vi "PXI_Host_I16_Write_NewMethod_Benchmark.vi"() -> ()   [LabVIEW 2018]
uses:
  <vilib>/Platform/TimedLoop/XDataNode/timing_clust.ctl
  <vilib>/Platform/TimedLoop/XDataNode/nitl_modes.ctl
  <vilib>/Platform/TimedLoop/XDataNode/wakeup.ctl
  cRIO RT/FPGA Bitfile Register Operations/Scalar IO Operations/Write Methods/Write Data Register/Instances/Write I16.vi
  cRIO RT/FPGA Bitfile Register Operations/Scalar IO Operations/Utilities/Find Register Offset.vi
  cRIO RT/FPGA Bitfile Register Operations/Scalar IO Operations/SubVIs/Check Register Data Store.vi
  cRIO RT/FPGA Bitfile Register Operations/Scalar IO Operations/Error Handling/Error 6001.vi
  cRIO RT/FPGA Bitfile Register Operations/Scalar IO Operations/Error Handling/Error 6000.vi
  cRIO RT/FPGA Bitfile Register Operations/Scalar IO Operations/Error Handling/Error 6002.vi
  cRIO RT/FPGA Bitfile Register Operations/Scalar IO Operations/Error Handling/Error 6006.vi
  <vilib>/FPGAPlugInAG/Dynamic/niLvFpga_Close_Dynamic.vi
  <vilib>/platform/TimedLoop/XDataNode/XDataNode.xnode
  <vilib>/rvi/interface/nirviCloseFPGA/nirviCloseFPGA.xnode
  cRIO RT/FPGA Bitfile Register Operations/Scalar IO Operations/FPGA Register IO.lvlib
  <vilib>/Platform/TimedLoop/XDataNode/XDNodeRunTimeDep.lvlib
panel:
  out "Maximum(s)":dbl
  out "Standard deviation":dbl
  out "Waveform Graph":dbl[](graph)
  out "error out":errorcluster
  out "Execution time (s)":dbl
  # "Recorded time"
  # "3.37551E-5"
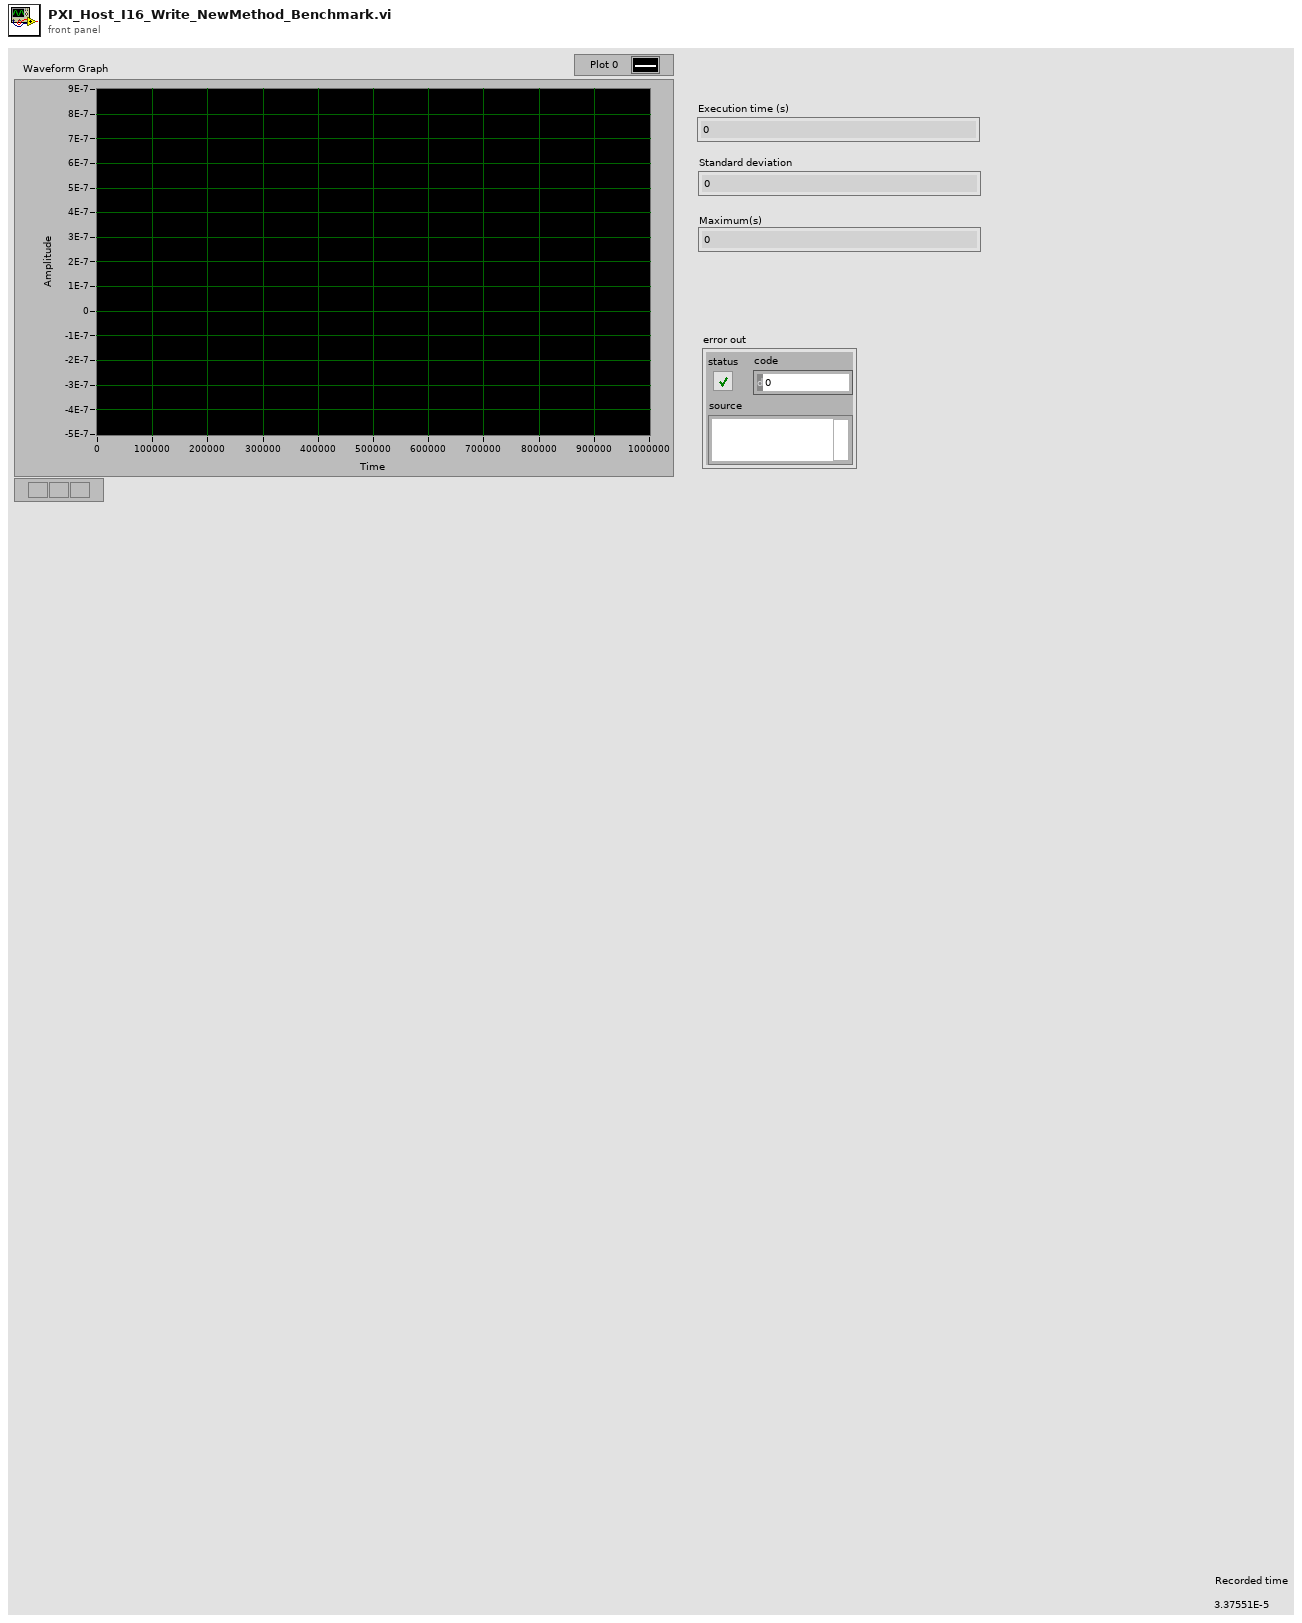
[diagram p1: front panel]
types:
  T1 = typedef "XDNodeRunTimeDep.lvlib/timing_clust.ctl" = cluster{"Expected End [f-1]":u64, "Actual End [f-1]":u64, "Finished Late? [f-1]":bool, "Expected End [i-1]":u64, "Actual End [i-1]":u64, "Finished Late? [i-1]":bool, "Expected Start [i]":u64, "Actual Start [i]":u64, "Expected Start [f]":u64, "Actual Start [f]":u64, "Source Name":string, "Structure Name":string, "Period":i64, "Deadline":i64, "Offset":i64, "Start":i64, "Priority":i32, "Timeout":i32, "Mode":T2, "Wakeup Reason":T3, "Error":errorcluster, "Source Type":string, "Secondary Source Type":string, "Global End Time":u64, "Global Start Time":u64, "Frame Duration":u64, "Iteration Duration":u64, "Assigned CPU":i32, "I/O Scan Engine Mode":u32}
  T2 = typedef "XDNodeRunTimeDep.lvlib/nitl_modes.ctl" = enum32{"No Change", "Process missed periods, maintain original phase", "Discard missed periods, maintain original phase", "Process missed periods, ignore original phase", "Discard missed periods, ignore original phase"}
  T3 = typedef "XDNodeRunTimeDep.lvlib/wakeup.ctl" = enum32{"Normal", "Aborted", "Asynchronous wakeup", "Timing source error", "Timed loop error", "Timeout"}
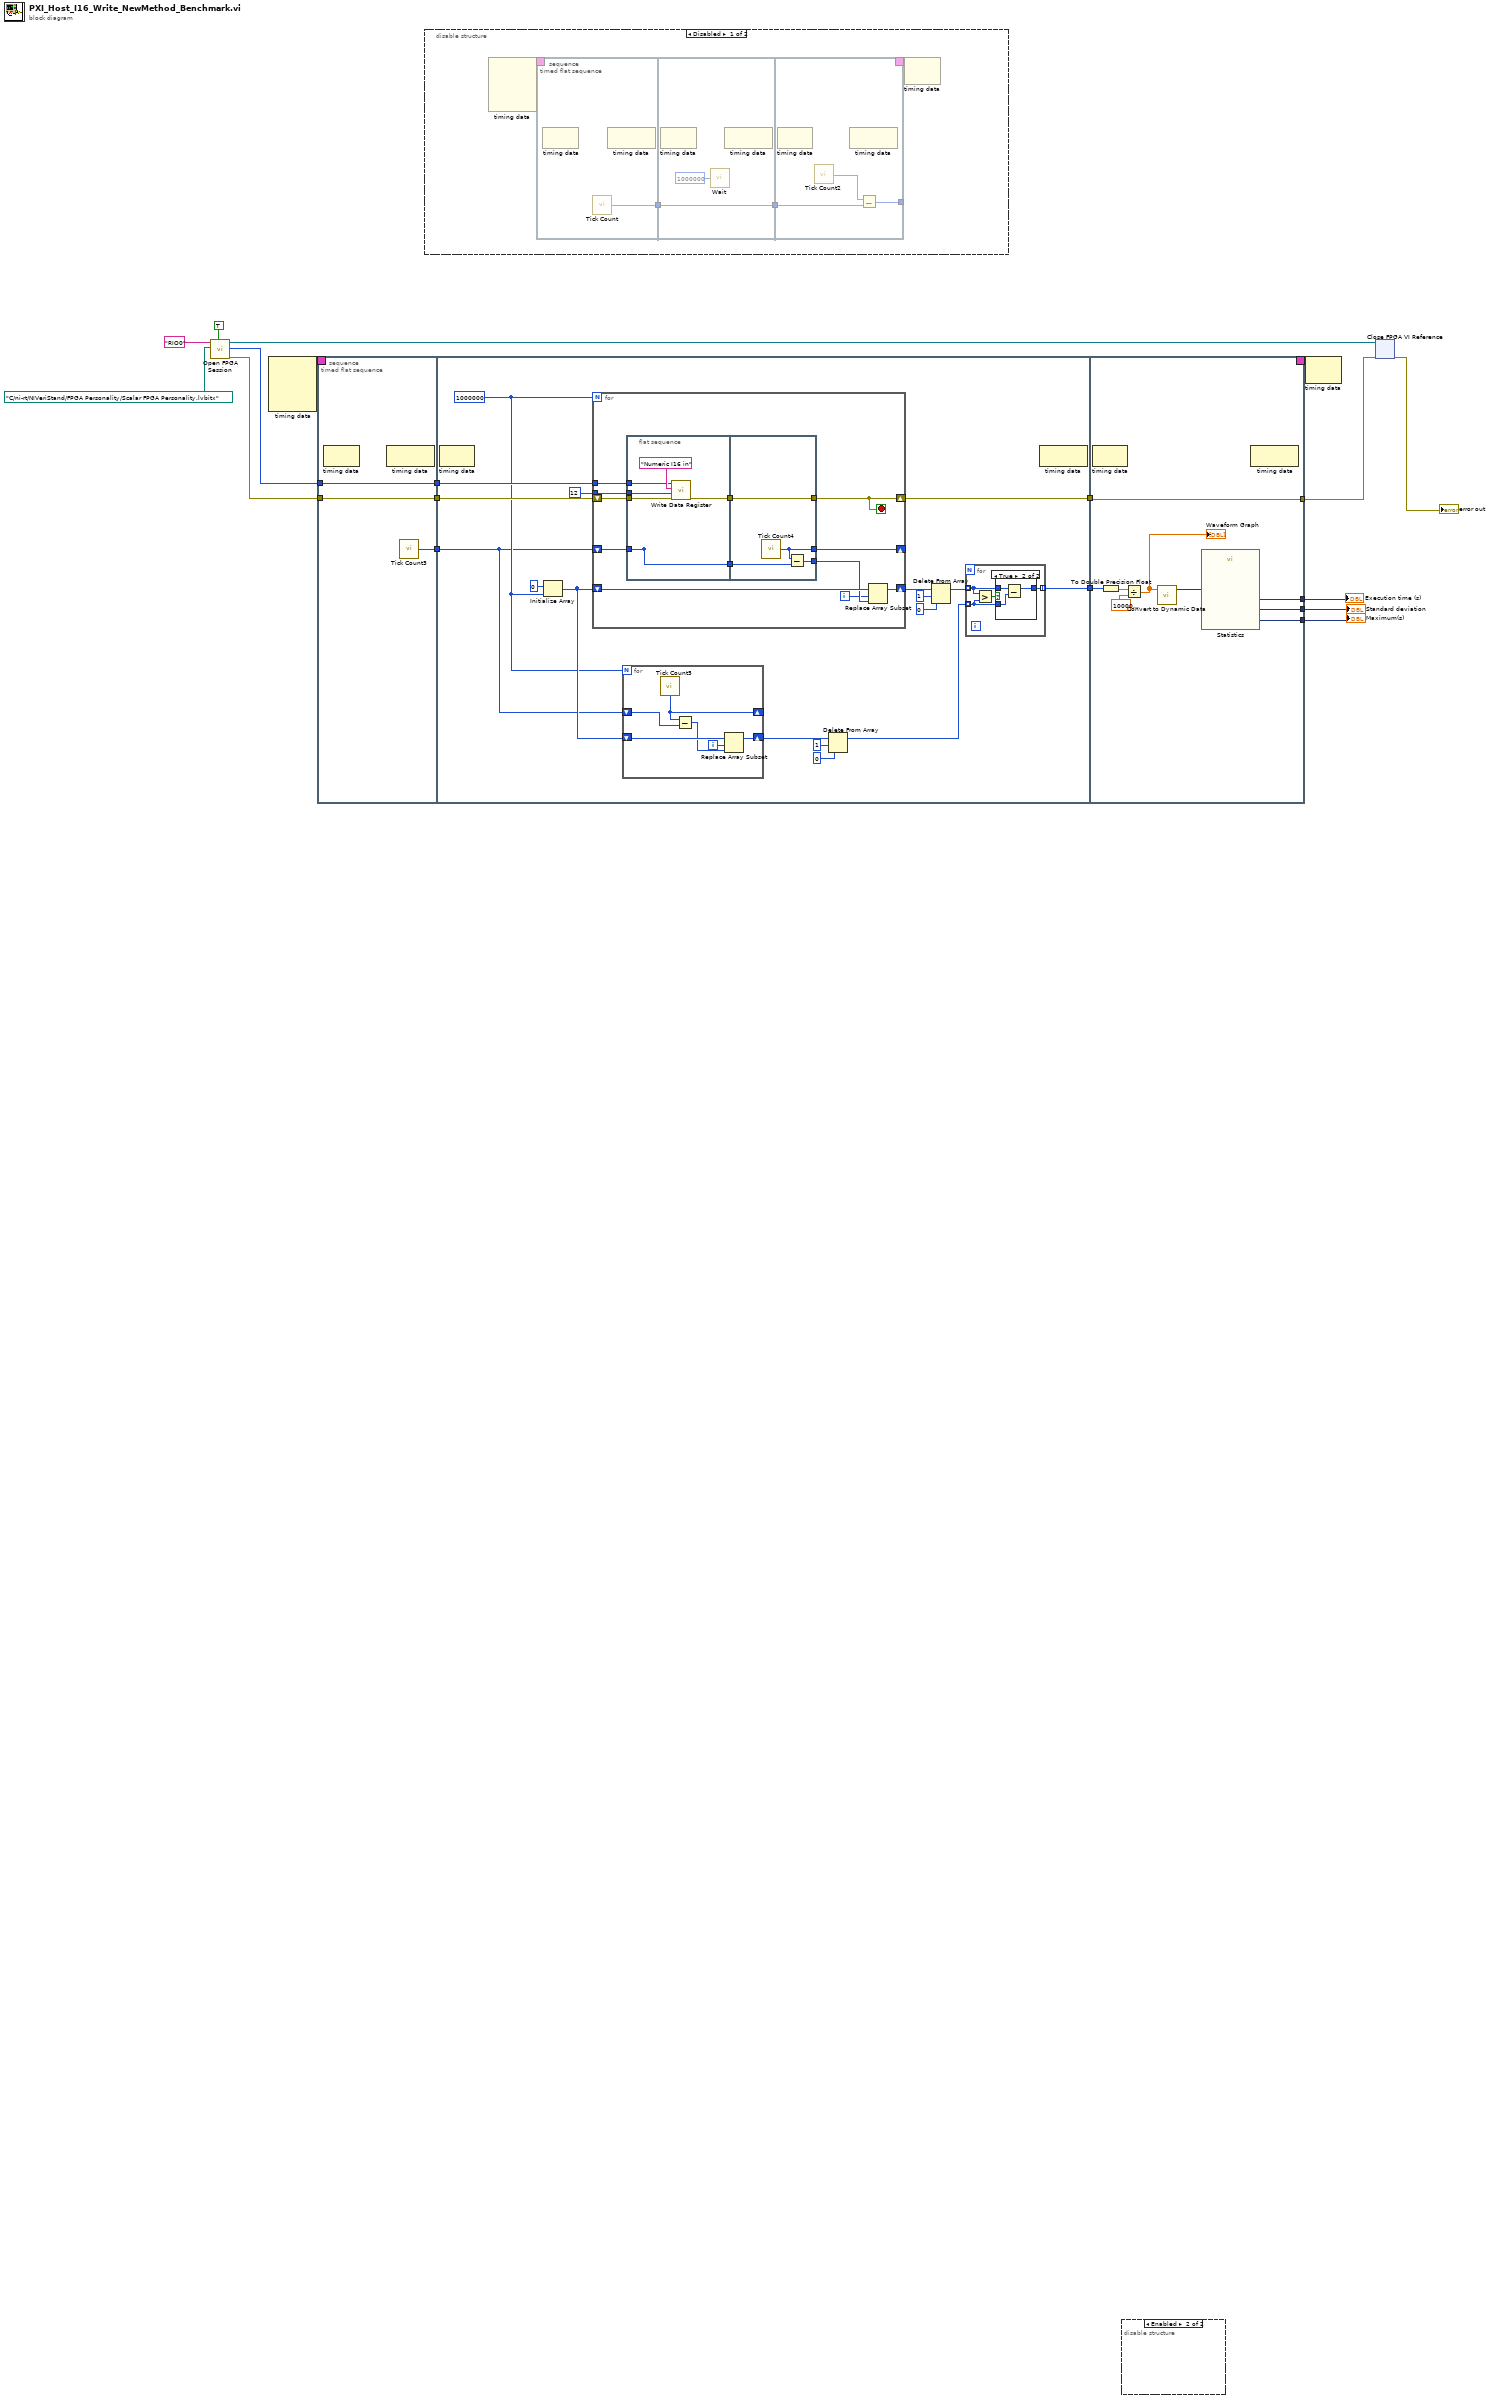
[diagram p0: block diagram]
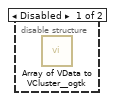
[diagram p4: hidden frame]
diagram:
  n1 = call "Open FPGA Session.vi"("run when loaded (T)"=TRUE, "bitfile path"=path "C:/ni-rt/NIVeriStand/FPGA Personality/Scalar FPGA Personality.lvbitx", "device address"="RIO0") -> ("error out"=w7:errorcluster, "session out"=w11:u32, "bitfile reference out"=w6:refnum<k20>)  [unwired: 6 in]
  n2 = node-c288() -> (w13:T1)  [unwired: 4 in]
  n3 = timed-sequence {
    timing: w13 -> [_]
    timing-out: [_] -> w12
    tunnel: w11 -> [w24]
    tunnel: w7 -> [w23]
    tunnel: [w19] -> w5
    tunnel: [w17] -> w3
    tunnel: [w16] -> w2
    tunnel: [w15] -> w1
    n4 = timed-flat-sequence {
      tunnel: w24 -> [w27]
      tunnel: [w27] -> w22
      tunnel: w23 -> [w26]
      tunnel: [w26] -> w21
      tunnel: [w25] -> w18
      tunnel: w22 -> [w46]
      tunnel: w21 -> [w45]
      tunnel: [w44] -> w20
      tunnel: w18 -> [w33]
      tunnel: [w30] -> w14
      tunnel: w20 -> [w93]
      tunnel: [w93] -> w19
      tunnel: [w91] -> w17
      tunnel: [w89] -> w16
      tunnel: [w88] -> w15
      tunnel: w14 -> [w86]
      frame #0 {
        n5 = node-c288() -> ()  [unwired: 1 in, 1 out]
        n6 = node-c288() -> ()  [unwired: 1 in, 1 out]
        n7 = call "Tick Count3"() -> ("Tick Count(Ticks)"=w25:u32)
      }
      frame #1 {
        w34 = 1000000
        n8 = node-c288() -> ()  [unwired: 1 in, 1 out]
        n9 = Initialize Array(0, w34) -> (w35:i32[])
        n10 = for {
          N: w34 -> [_]
          tunnel: w46 -> [w73]
          shift-right: [w71] -> _
          shift-left: w33 -> [w70]
          shift-right: [w66] -> w43
          shift-left: w35 -> [w68]
          shift-right: [w64] -> w44
          shift-left: w45 -> [w74]
          tunnel: i16 12 ("value in") -> [w63]
          i -> [w65]
          stop <- w64 stop-if-true
          n11 = flat-sequence {
            tunnel: w74 -> [w78]
            tunnel: w73 -> [w75]
            tunnel: [w77] -> w72
            tunnel: [w80] -> _
            tunnel: w70 -> [w80]
            tunnel: [w80] -> w69
            tunnel: w63 -> [w76]
            tunnel: [w84] -> w64
            tunnel: w72 -> [w84]
            tunnel: [w81] -> w71
            tunnel: w69 -> [w83]
            tunnel: [w82] -> w67
            frame #0 {
              n12 = call-poly "Write Data Register.vi"("error in"=w78, "value in"=w76, "register name"="Numeric I16 in", "session in"=w75) -> ("error out"=w77:errorcluster)  [unwired: 6 in, 1 out]
            }
            frame #1 {
              n13 = call "Tick Count4"() -> ("Tick Count(Ticks)"=w81:u32)
              n14 = Subtract(x=w81, y=w83) -> (x-y=w82:u32)
            }
          }
          n15 = Replace Array Subset(array=w68, new element=w67, index=w65) -> (w66:i32[])
        }
        n16 = for {
          N: w34 -> [_]
          shift-right: [w55] -> w36
          shift-left: w35 -> [w58]
          shift-right: [w60] -> _
          shift-left: w33 -> [w59]
          i -> [w56]
          n17 = call "Tick Count5"() -> ("Tick Count(Ticks)"=w60:u32)
          n18 = Subtract(x=w60, y=w59) -> (x-y=w57:u32)
          n19 = Replace Array Subset(array=w58, new element=w57, index=w56) -> (w55:i32[])
        }
        n20 = Delete From Array(array=w36, length=1, index=0) -> (array with subset deleted=w31:i32[])  [unwired: 1 out]
        n21 = Delete From Array(array=w43, length=1, index=0) -> (array with subset deleted=w32:i32[])  [unwired: 1 out]
        n22 = for {
          tunnel: [w50] -> w30 mode=indexing
          tunnel: w32 -> [w49] mode=indexing
          tunnel: w31 -> [w48] mode=indexing
          n23 = Greater?(x=w49, y=w48) -> (0:w47:bool)
          n24 = case shown="True" w47 {
            tunnel: w49 -> [w51 w54]
            tunnel: w48 -> [_ w53]
            tunnel: [w51 w52] -> w50
            frame False {
            }
            frame True {
              n25 = Subtract(x=w54, y=w53) -> (x-y=w52:i32)
            }
          }
        }
        n26 = node-c288() -> ()  [unwired: 1 in, 1 out]
      }
      frame #2 {
        n27 = node-c288() -> ()  [unwired: 1 in, 1 out]
        n28 = To Double Precision Float(number=w86) -> (double precision float=w87:dbl[])
        n29 = Divide(x=w87, y=1000000000.0) -> (x/y=w85:dbl[])
        "Waveform Graph" <- w85
        n30 = call "Convert to Dynamic Data"("Array"=w85) -> ("Dynamic Data Type"=w92:dynamicdata)  [unwired: 3 in]
        n31 = call "Statistics"("Signals"=w92) -> ("Standard Dev"=w89:dynamicdata, "Arithmetic Mean"=w91:dynamicdata, "Maximum"=w88:dynamicdata)  [unwired: 23 in, 1 out]
        n32 = node-c288() -> ()  [unwired: 1 in, 1 out]
      }
    }
  }
  "Execution time (s)" <- w3
  "Standard deviation" <- w2
  "Maximum(s)" <- w1
  n33 = disable-structure shown="Disabled" {
    frame Disabled {
      n34 = node-c288() -> (w97:T1)  [unwired: 4 in]
      n35 = timed-sequence {
        timing: w97 -> [_]
        timing-out: [_] -> w96
        tunnel: [w98] -> _
        n36 = timed-flat-sequence {
          tunnel: [w101] -> w100
          tunnel: w100 -> [w104]
          tunnel: [w104] -> w99
          tunnel: w99 -> [w110]
          tunnel: [w108] -> w98
          frame #0 {
            n37 = node-c288() -> ()  [unwired: 1 in, 1 out]
            n38 = call "Tick Count"() -> ("Tick Count(Ticks)"=w101:u32)
            n39 = node-c288() -> ()  [unwired: 1 in, 1 out]
          }
          frame #1 {
            n40 = node-c288() -> ()  [unwired: 1 in, 1 out]
            n41 = call "Wait"("Count(uSec)"=u32 1000000 ("Count(mSec)")) -> ()  [unwired: 1 out]
            n42 = node-c288() -> ()  [unwired: 1 in, 1 out]
          }
          frame #2 {
            n43 = node-c288() -> ()  [unwired: 1 in, 1 out]
            n44 = call "Tick Count2"() -> ("Tick Count(Ticks)"=w109:u32)
            n45 = node-c288() -> ()  [unwired: 1 in, 1 out]
            n46 = Subtract(x=w109, y=w110) -> (x-y=w108:u32)
          }
        }
      }
      n47 = node-c288(w96) -> ()  [unwired: 1 out]
    }
    frame Enabled {
    }
  }
  n48 = disable-structure shown="Enabled" {
    frame Disabled {
      n49 = call <userlib>:"Array of VData to VCluster__ogtk.vi"() -> ()  [unwired: 10 in, 2 out]
    }
    frame Enabled {
    }
  }
  n50 = node-c288(w12) -> ()  [unwired: 1 out]
  n51 = xnode "Close FPGA VI Reference"("FPGA VI Reference In"=w6, "error in"=w5) -> ("error out"=→"error out":errorcluster)
